vi "empty.vi"(8 "errorIn":errorcluster, 11 "refer":refnum<queue>) -> (0 "errorOut":errorcluster, 3 "refer":refnum<queue>)   [LabVIEW 2017]
uses:
  models/EMSGData.ctl
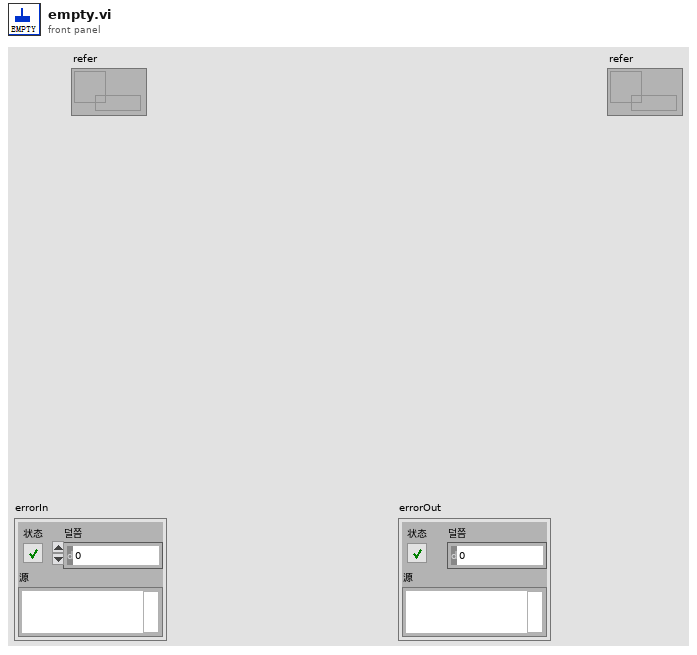
[diagram p1: front panel]
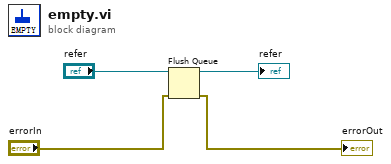
[diagram p0: block diagram]
diagram:
  n1 = Flush Queue(queue="refer", error in (no error)="errorIn") -> (queue out=→"refer":refnum<queue>, error out=→"errorOut":errorcluster)  [unwired: 1 out]
